vi "TCP Command Sent.vi"(6 "Message":string, 8 "error in (no error)":errorcluster, 9 "Sending Error":errorcluster, 10 "GUID":string, 11 "tWorkerController in":refnum<class "tWorkerController.lvclass">) -> (0 "error out":errorcluster, 3 "tWorkerController out":refnum<class "tWorkerController.lvclass">)   [LabVIEW 2013, in "tWorkerController.lvlib" / "tWorkerController.lvclass"]
uses:
  tWorkerController.lvclass
  <vilib>/ActorFramework/Actor/Actor.lvclass/Actor.ctl
  LVAutomationListener/msgs/Log Event Msg/Log Event Msg.lvclass/Log Event Msg.ctl
  <vilib>/ActorFramework/Message Enqueuer/Message Enqueuer.lvclass/Message Enqueuer.ctl
  <vilib>/Utility/error.llb/DialogType.ctl
  <vilib>/ActorFramework/Message Enqueuer/Enqueue.vi
  <vilib>/ActorFramework/Message Priority Queue/Priority Enqueue.vi
  LVAutomationListener/msgs/Log Event Msg/Log Event Msg.lvclass
  <vilib>/ActorFramework/Actor/Actor.lvclass
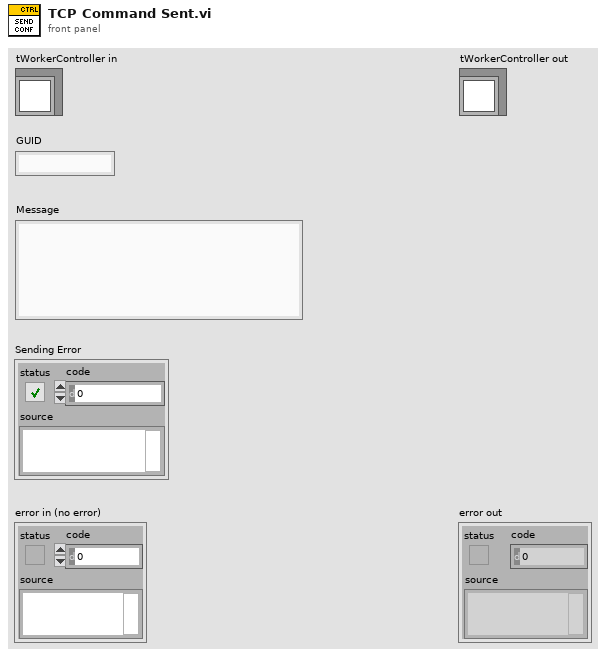
[diagram p1: front panel]
types:
  T1 = typedef "DialogType.ctl" = u16
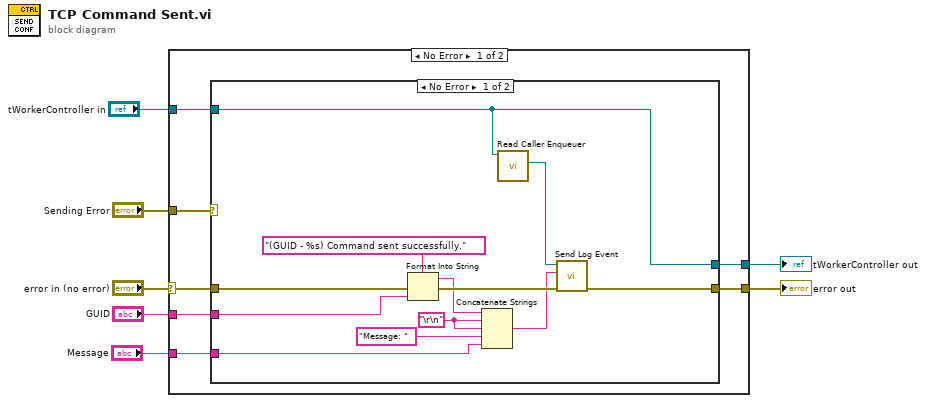
[diagram p0: block diagram]
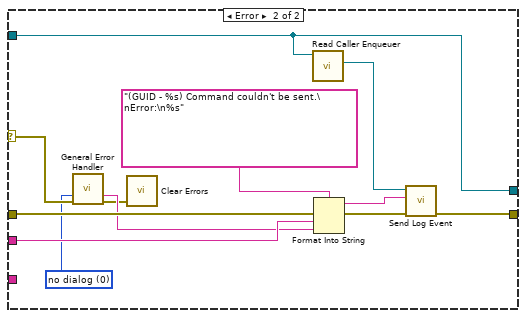
[diagram p2: hidden frame]
diagram:
  n1 = case shown="No Error" "error in (no error)" {
    selector: "error in (no error)" -> [w10 w40]
    tunnel: [w12 w40] -> w6
    tunnel: [w14 w39] -> w4
    tunnel: "tWorkerController in" -> [w9 w39]
    tunnel: "GUID" -> [w11 _]
    tunnel: "Sending Error" -> [w13 _]
    tunnel: "Message" -> [w8 _]
    frame No Error {
      n2 = case shown="No Error" w13 {
        selector: w13 -> [_ w30]
        tunnel: w10 -> [w26 w34]
        tunnel: w9 -> [w21 w31]
        tunnel: [w20 w32] -> w12
        tunnel: [w21 w31] -> w14
        tunnel: w11 -> [w24 w33]
        tunnel: w8 -> [w15 _]
        frame No Error {
          w16 = "\r\n"
          n3 = Format Into String(format string="(GUID - %s) Command sent successfully.", error in=w26, w24) -> (resulting string=w19:string, error out=w23:errorcluster)  [unwired: 1 in]
          n4 = Concatenate Strings(w19, w16, w16, "Message: " ("string"), w15) -> (w18:string)
          n5 = call <vilib>:"Read Caller Enqueuer.vi"("Actor"=w21) -> ("Caller Enqueuer"=w22:refnum<class "Message Enqueuer.lvclass">)  [unwired: 10 in]
          n6 = call "Send Log Event.vi"("error in (no error)"=w23, "Event Text"=w18, "Message Enqueuer"=w22) -> ("error out"=w20:errorcluster)  [unwired: 7 in, 1 out]
        }
        frame Error {
          w28 = T1 0 items=["no dialog", "OK message", "continue or stop message", "OK message + warnings", "continue/stop + warnings"] ("type of dialog (OK msg:1)")
          n7 = call <vilib>:"General Error Handler.vi"("type of dialog (OK msg:1)"=w28, "error in (no error)"=w30) -> ("message"=w29:string, "error out"=w27:errorcluster)  [unwired: 9 in, 3 out]
          n8 = call <vilib>:"Clear Errors.vi"("error in (no error)"=w27) -> ()  [unwired: 6 in, 1 out]
          n9 = call <vilib>:"Read Caller Enqueuer.vi"("Actor"=w31) -> ("Caller Enqueuer"=w38:refnum<class "Message Enqueuer.lvclass">)  [unwired: 10 in]
          n10 = Format Into String(format string="(GUID - %s) Command couldn't be sent.\nError:\n%s", error in=w34, w33, w29) -> (resulting string=w37:string, error out=w36:errorcluster)  [unwired: 1 in]
          n11 = call "Send Log Event.vi"("error in (no error)"=w36, "Event Text"=w37, "Message Enqueuer"=w38) -> ("error out"=w32:errorcluster)  [unwired: 7 in, 1 out]
        }
      }
    }
    frame Error {
    }
  }
  "error out" <- w6
  "tWorkerController out" <- w4
